vi "Test ASCII settings.vi"() -> ()   [LabVIEW 2015]
panel:
  in  "Array 3":dbl[](array[numeric])
  out "Boolean":bool
  in  "Numeric 2":i32
  in  "Path":path
  out "Array 2":string[](array[string])
  out "Array":u32[](array[numeric])
  in  "String":string
  in  "Numeric":dbl
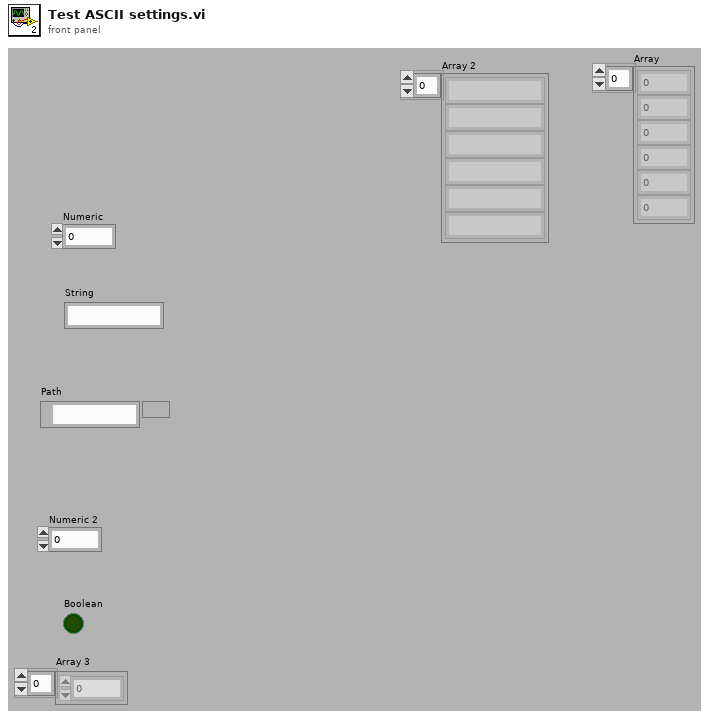
[diagram p1: front panel]
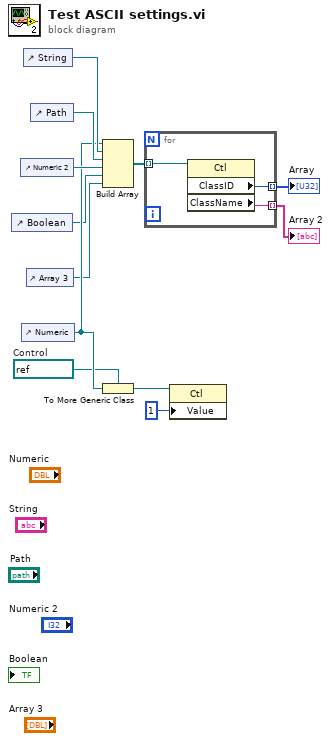
[diagram p0: block diagram]
diagram:
  w5 = refnum<vi> refnum  # Control
  n1 = control-ref of="Boolean"() -> (w2:refnum<vi>)
  n2 = control-ref of="Numeric 2"() -> (w7:refnum<vi>)
  n3 = control-ref of="Numeric"() -> (w6:refnum<vi>)
  n4 = control-ref of="String"() -> (w12:refnum<vi>)
  n5 = control-ref of="Array 3"() -> (w1:refnum<vi>)
  n6 = control-ref of="Path"() -> (w8:refnum<vi>)
  n7 = Build Array(w6, w12, w8, w7, w2, w1) -> (w11:refnum<vi>[])
  n8 = To More Generic Class(target class=w5, reference=w6) -> (generic class reference=w4:refnum<vi>)
  n9 = for {
    tunnel: w11 -> [w15] mode=indexing
    tunnel: [w14] -> w10 mode=indexing
    tunnel: [w13] -> w9 mode=indexing
    n10 = property class="Ctl"(reference=w15) -> ("ClassID"=w14:u32, "ClassName"=w13:string)  [unwired: 1 in, 2 out]
  }
  "Array" <- w10
  "Array 2" <- w9
  n11 = property class="Ctl"(reference=w4, "Value"=1) -> ()  [unwired: 1 in, 2 out]
